vi "Get_Timer.vi"(8 "error in (no error)":errorcluster, 11 "Timer_Event in":refnum<class "Timer_Event.lvclass">) -> (0 "error out":errorcluster, 1 "Running":bool, 2 "Elapsed Time (ms)":u32, 3 "Timer_Event out":refnum<class "Timer_Event.lvclass">)   [LabVIEW 2020, in "Timer_Event.lvlib" / "Timer_Event.lvclass"]
uses:
  Timer_Event.lvclass
  Timer_Event.lvclass/Timer_Event.ctl
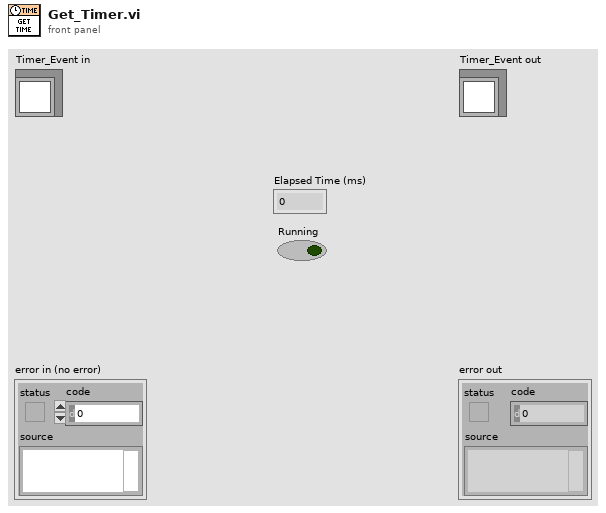
[diagram p1: front panel]
types:
  T1 = cluster{"Start Time":i32, "Elapsed Time":i32, "Running?":bool}
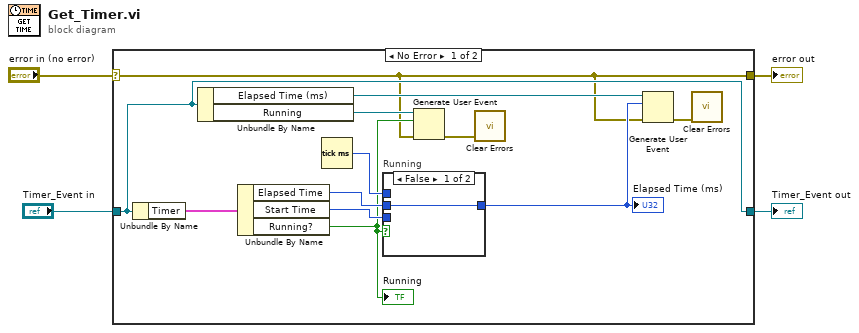
[diagram p0: block diagram]
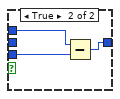
[diagram p2: hidden frame]
diagram:
  n1 = case shown="No Error" "error in (no error)" {
    selector: "error in (no error)" -> [w7 w22]
    tunnel: [w7 w22] -> w3
    tunnel: [w12 w21] -> w1
    tunnel: "Timer_Event in" -> [w12 w21]
    frame No Error {
      n2 = Unbundle By Name(w12) -> ("Timer"=w13:T1)
      n3 = Unbundle By Name(w12) -> ("Elapsed Time (ms)"=w11:refnum<user-event>, "Running"=w9:refnum<user-event>)
      n4 = Unbundle By Name(w13) -> ("Elapsed Time"=w16:i32, "Start Time"=w15:i32, "Running?"=w8:bool)
      "Running" <- w8
      n5 = Tick Count (ms)() -> (millisecond timer value=w14:u32)
      n6 = case "Running" shown="False" w8 {
        tunnel: w14 -> [_ w20]
        tunnel: w15 -> [_ w19]
        tunnel: [w17 w18] -> w10
        tunnel: w16 -> [w17 _]
        frame False {
        }
        frame True {
          n7 = Subtract(x=w20, y=w19) -> (x-y=w18:u32)
        }
      }
      "Elapsed Time (ms)" <- w10
      n8 = Generate User Event(user event=w9, event data cluster=w8, error in=w7) -> (error out=w6:errorcluster)  [unwired: 1 in, 1 out]
      n9 = call <vilib>:"Clear Errors.vi"("error in (no error)"=w6) -> ()  [unwired: 5 in, 2 out]
      n10 = Generate User Event(user event=w11, event data cluster=w10, error in=w7) -> (error out=w5:errorcluster)  [unwired: 1 in, 1 out]
      n11 = call <vilib>:"Clear Errors.vi"("error in (no error)"=w5) -> ()  [unwired: 5 in, 2 out]
    }
    frame Error {
    }
  }
  "error out" <- w3
  "Timer_Event out" <- w1
